vi "SDCP TMC Decode.vi"(2 "error in (no error)":errorcluster, 3 "Frame":u8[](array[numeric])) -> (0 "error out":errorcluster, 1 "SDCP TMC out":T1)   [LabVIEW 2020]
uses:
  Typedefs/SDCP TMC Param.ctl
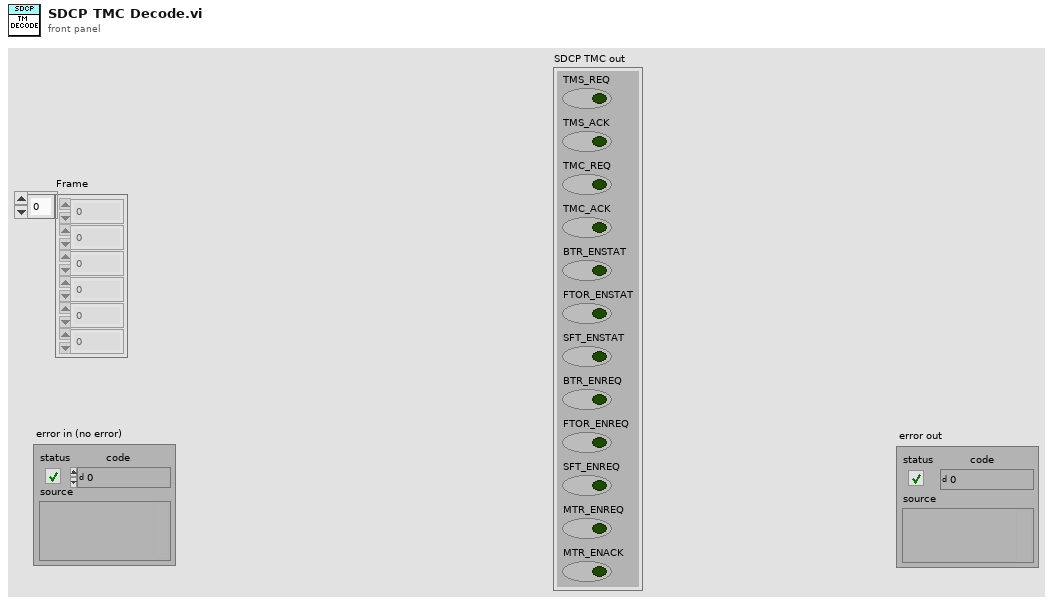
[diagram p1: front panel]
types:
  T1 = typedef "SDCP TMC Param.ctl" = cluster{"TMS_REQ":bool, "TMS_ACK":bool, "TMC_REQ":bool, "TMC_ACK":bool, "BTR_ENSTAT":bool, "FTOR_ENSTAT":bool, "SFT_ENSTAT":bool, "BTR_ENREQ":bool, "FTOR_ENREQ":bool, "SFT_ENREQ":bool, "MTR_ENREQ":bool, "MTR_ENACK":bool}
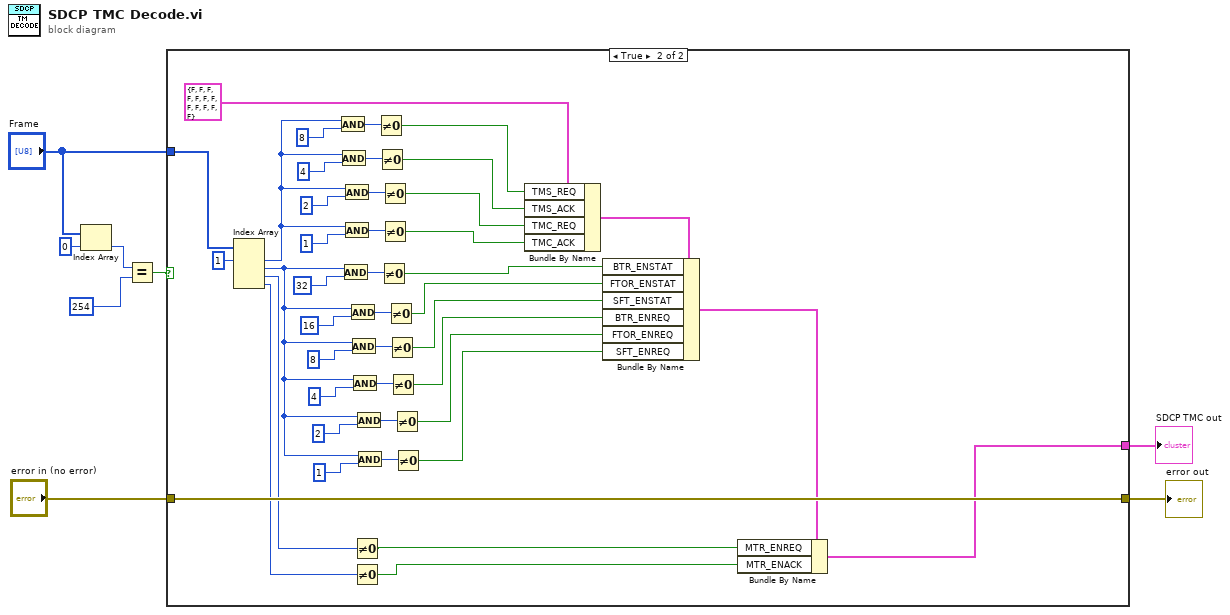
[diagram p0: block diagram]
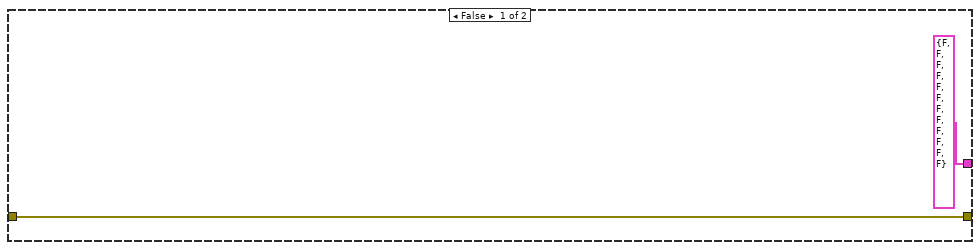
[diagram p2: hidden frame]
diagram:
  n1 = Index Array(array="Frame", index=0) -> (element=w7:u8)
  n2 = Equal?(x=w7, y=u8 254) -> (x = y?=w5:bool)
  n3 = case shown="True" w5 {
    tunnel: "error in (no error)" -> [w10 w53]
    tunnel: [w10 w53] -> w3
    tunnel: "Frame" -> [_ w52]
    tunnel: [T1 {"TMS_REQ"=FALSE, "TMS_ACK"=FALSE, "TMC_REQ"=FALSE, "TMC_ACK"=FALSE, "BTR_ENSTAT"=FALSE, "FTOR_ENSTAT"=FALSE, "SFT_ENSTAT"=FALSE, "BTR_ENREQ"=FALSE, "FTOR_ENREQ"=FALSE, "SFT_ENREQ"=FALSE, "MTR_ENREQ"=FALSE, "MTR_ENACK"=FALSE} ("SDCP TMC Param") w43] -> w1
    frame False {
    }
    frame True {
      n4 = Index Array(array=w52, index #1=1 ("index")) -> (element #1=w31:u8, element #2=w12:u8, element #3=w48:u8, element #4=w47:u8)  [unwired: 3 in]
      n5 = And(x=w31, y=u8 8) -> (x .and. y?=w41:u8)
      n6 = And(x=w31, y=u8 4) -> (x .and. y?=w38:u8)
      n7 = And(x=w12, y=u8 32) -> (x .and. y?=w28:u8)
      n8 = And(x=w31, y=u8 2) -> (x .and. y?=w35:u8)
      n9 = And(x=w31, y=u8 1) -> (x .and. y?=w32:u8)
      n10 = And(x=w12, y=u8 16) -> (x .and. y?=w25:u8)
      n11 = And(x=w12, y=u8 8) -> (x .and. y?=w22:u8)
      n12 = And(x=w12, y=u8 4) -> (x .and. y?=w19:u8)
      n13 = Not Equal To 0?(x=w48) -> (x != 0?=w45:bool)
      n14 = Not Equal To 0?(x=w47) -> (x != 0?=w44:bool)
      n15 = And(x=w12, y=u8 2) -> (x .and. y?=w16:u8)
      n16 = And(x=w12, y=u8 1) -> (x .and. y?=w13:u8)
      n17 = Not Equal To 0?(x=w41) -> (x != 0?=w40:bool)
      n18 = Not Equal To 0?(x=w38) -> (x != 0?=w37:bool)
      n19 = Not Equal To 0?(x=w28) -> (x != 0?=w27:bool)
      n20 = Not Equal To 0?(x=w35) -> (x != 0?=w34:bool)
      n21 = Not Equal To 0?(x=w32) -> (x != 0?=w30:bool)
      n22 = Not Equal To 0?(x=w25) -> (x != 0?=w24:bool)
      n23 = Not Equal To 0?(x=w22) -> (x != 0?=w21:bool)
      n24 = Not Equal To 0?(x=w19) -> (x != 0?=w18:bool)
      n25 = Not Equal To 0?(x=w16) -> (x != 0?=w15:bool)
      n26 = Not Equal To 0?(x=w13) -> (x != 0?=w11:bool)
      n27 = Bundle By Name(cluster=T1 {"TMS_REQ"=FALSE, "TMS_ACK"=FALSE, "TMC_REQ"=FALSE, "TMC_ACK"=FALSE, "BTR_ENSTAT"=FALSE, "FTOR_ENSTAT"=FALSE, "SFT_ENSTAT"=FALSE, "BTR_ENREQ"=FALSE, "FTOR_ENREQ"=FALSE, "SFT_ENREQ"=FALSE, "MTR_ENREQ"=FALSE, "MTR_ENACK"=FALSE} ("SDCP TMC Param"), "TMS_REQ"=w40, "TMS_ACK"=w37, "TMC_REQ"=w34, "TMC_ACK"=w30) -> (w49:T1)
      n28 = Bundle By Name(cluster=w49, "BTR_ENSTAT"=w27, "FTOR_ENSTAT"=w24, "SFT_ENSTAT"=w21, "BTR_ENREQ"=w18, "FTOR_ENREQ"=w15, "SFT_ENREQ"=w11) -> (w46:T1)
      n29 = Bundle By Name(cluster=w46, "MTR_ENREQ"=w45, "MTR_ENACK"=w44) -> (w43:T1)
    }
  }
  "error out" <- w3
  "SDCP TMC out" <- w1
